vi "Insight_Reduce_Data_with_Valid-Vector.vi"(8 "error in (no error)":errorcluster, 9 "Valid Vector":i32[](array[numeric]), 11 "Raw Data":dbl[](array[numeric])) -> (0 "error out":errorcluster, 3 "Valid Data":dbl[](array[numeric]))   [LabVIEW 2010]
doc: "Insight Photonic Solutions\n\nver 1.0 - original release\n\nThis VI inputs raw data from an acquisition with the laser and outputs Valid Data, that is cleaned of the hold points in the sweep (sporadically during a sweep). The valid data are located at indices given by the \"Valid Vector\".\n\nHow to use this VI:\n1. After a sweep calibration is performed, request the Indices of the Invalid Data Points from the laser. These indices will be correct until the next time a sweep calibration is performed.\n\n2. Construct the Valid Vector, using \"Insight_Create_Valid_Vector.vi\", before beginning a data acquisition sequence. You only need to do this once, right after the sweep calibration. This saves time in data processing and allows the data to flow quickly from the Data Acquisition card to your image processing code.\n\n3. For each data acquisition, send the Raw Data from the Data Acquisition card to this vi \"Insight_Reduce_Data_with_Valid-Vector.vi\".\n\n4. Send the \"Valid Data\" to your image processing software."
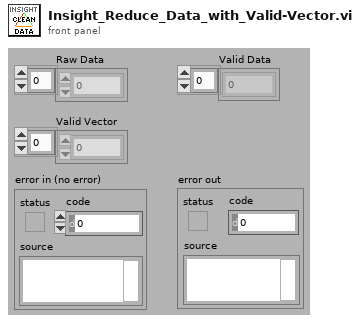
[diagram p1: front panel]
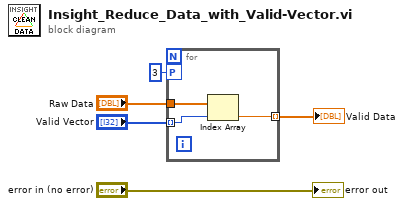
[diagram p0: block diagram]
diagram:
  n1 = for {
    tunnel: "Raw Data" -> [w8]
    tunnel: "Valid Vector" -> [w7] mode=indexing
    tunnel: [w6] -> w1 mode=indexing
    workers-P: 3 -> [_]
    n2 = Index Array(array=w8, index=w7) -> (element=w6:dbl)
  }
  "Valid Data" <- w1
  "error out" <- "error in (no error)"
